vi "motor safety.vi"(0 "Desired Rate":dbl, 1 "Forward Limit":dbl, 2 "Reverse Limit":dbl, 3 "Cutoff Rate":dbl=0.2, 4 "Max Rate":dbl=50.0, 5 "Min Rate":dbl, 6 "Encoder Refnum":string) -> (7 "Encoder Disconnected":bool, 9 "No Rate Read":bool, 11 "At Distance Limit":bool, 13 "Encoder Directional Issue":bool, 14 "Rate Output":dbl)   [LabVIEW 2013]
doc: "This VI provides two types of safety for your motors. An encoder for the motor is required. If the encoder reference is innalid, the motor won't be allowed to run. \nThe first safetyis a distance limit. The forward and reverse limit parameters specify the max and min valus for the encoder distance to read until the motor is stopped and only allowed to move away from its limit. \nThe second safety is an encoder safety. The Cutoff Rate parameter is the maximum value allowed to be sent to the motor without a response seen from the encoder. So, if the code is trying to set a value higher than this parameter and the encoder doesn't register a response, the motor will be disabled. It will be reenabled when movement is registered from the encoder. This safety will also permanately disable the motor if the encoder reads some inanely high rate. Consider a replacement...."
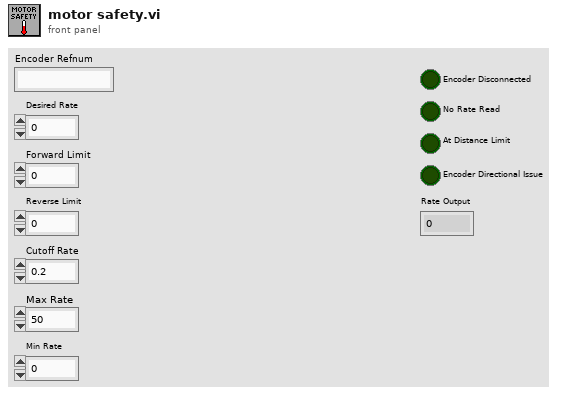
[diagram p1: front panel]
types:
  T1 = typedef "WPI_EncoderDevRef.ctl" = cluster{"DevStatus":errorcluster, "EncoderIndex":T2, "CounterIndex":T3, "DistancePerCount":dbl, "Decoding Type":T4}
  T2 = typedef "FPGA_EncoderIdx.ctl" = enum8{"Enc 0", "Enc 1", "Enc 2", "Enc 3", "Invalid"}
  T3 = typedef "FPGA_CounterCtrSystemIndex.ctl" = enum8{"Ctr 0", "Ctr 1", "Ctr 2", "Ctr 3", "Ctr 4", "Ctr 5", "Ctr 6", "Ctr 7", "Invalid"}
  T4 = typedef "WPI_EncoderType.ctl" = enum16{"1x", "2x", "4x"}
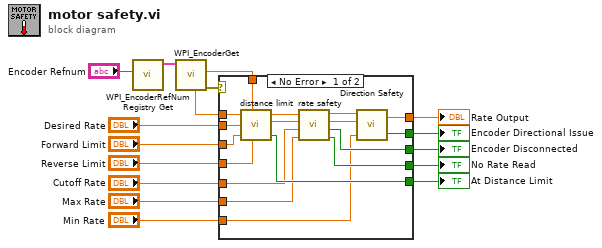
[diagram p0: block diagram]
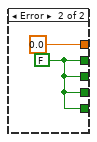
[diagram p2: hidden frame]
diagram:
  n1 = call <vilib>:"WPI_EncoderRefNum Registry Get.vi"("refnum name"="Encoder Refnum") -> ("EncoderDevRef"=w15:T1)  [unwired: 9 in, 1 out]
  n2 = call <vilib>:"WPI_EncoderGet.vi"("EncoderDevRef"=w15) -> ("error out"=w7:errorcluster, "Distance"=w12:dbl, "Rate"=w14:dbl)  [unwired: 5 in, 3 out]
  n3 = case shown="No Error" w7 {
    tunnel: w14 -> [w29 _]
    tunnel: "Desired Rate" -> [w28 _]
    tunnel: w12 -> [w26 _]
    tunnel: [w21 0.0 ("Output Rate")] -> w11
    tunnel: "Forward Limit" -> [w25 _]
    tunnel: "Reverse Limit" -> [w24 _]
    tunnel: "Cutoff Rate" -> [w20 _]
    tunnel: [w33 w34] -> w6
    tunnel: [w32 w34] -> w5
    tunnel: "Max Rate" -> [w18 _]
    tunnel: "Min Rate" -> [w17 _]
    tunnel: [w31 w34] -> w2
    tunnel: [w30 w34] -> w1
    frame No Error {
      n4 = call "distance limit.vi"("Encoder Rate"=w29, "Encoder Distance"=w26, "Desired Rate"=w28, "Forward Limit"=w25, "Reverse Limit"=w24) -> ("Encoder Rate Out"=w27:dbl, "Output Rate"=w19:dbl, "At Distance Limit"=w30:bool)
      n5 = call "rate safety.vi"("Max Rate"=w18, "Cutoff Rate"=w20, "Desired Rate"=w19, "Encoder Rate"=w27) -> ("No Rate Read"=w32:bool, "Encoder Disconnected"=w33:bool, "Output Rate"=w22:dbl, "Encoder Rate Out"=w23:dbl)
      n6 = call "Direction Safety.vi"("Min Rate"=w17, "Desired Rate"=w22, "Encoder Rate"=w23) -> ("Encoder Directional Issue"=w31:bool, "Super Safe Rate"=w21:dbl)
    }
    frame Error {
      w34 = FALSE ("Cutoff Tripped")
    }
  }
  "Rate Output" <- w11
  "Encoder Disconnected" <- w6
  "No Rate Read" <- w5
  "Encoder Directional Issue" <- w2
  "At Distance Limit" <- w1
